vi "Calculate Duty Cycle.vi"(0 "Voltage/Current Values":dbl[](array[numeric]), 5 "Pulse voltage/Current level":dbl=1.0, 7 "Sample rate":dbl, 9 "Frequency":dbl, 11 "error in":errorcluster) -> (4 "Duty Cycle":dbl, 15 "error out":errorcluster)   [LabVIEW 2021]
doc: "This VI calculates the duty cycle high percentage using the rising and falling thresholds of current/voltage vaules."
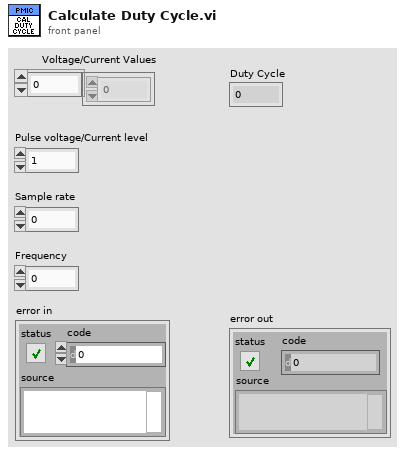
[diagram p1: front panel]
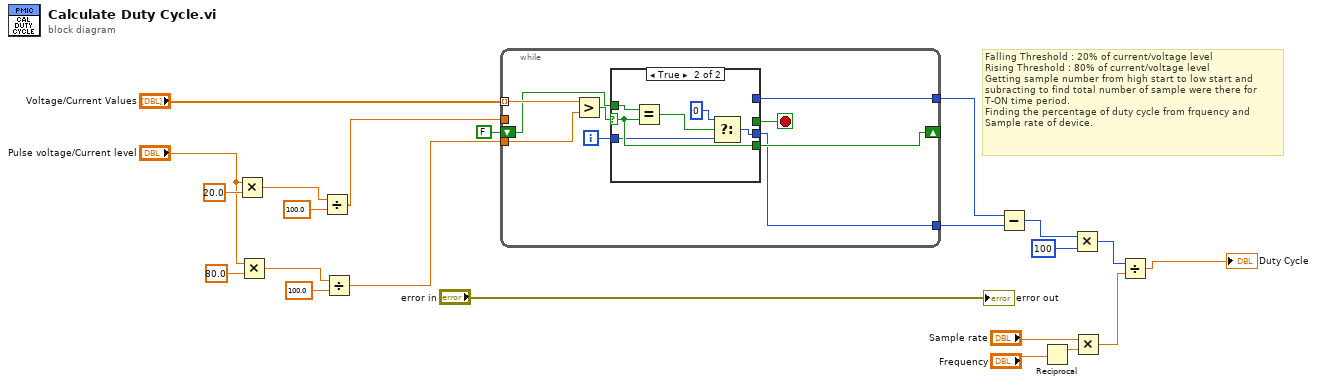
[diagram p0: block diagram]
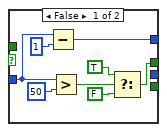
[diagram p2: hidden frame]
diagram:
  # "Falling Threshold : 20% of current/voltage level\nRising Threshold : 80% of current/voltage level\nGetting sample number from high start to low start and \nsubracting to find total number of sample were there for\nT-ON time period.\nFinding the percentage of duty cycle from frquency and\nSample rate of device."
  n1 = Multiply(x="Pulse voltage/Current level", y=20.0) -> (x*y=w21:dbl)
  n2 = Multiply(x="Pulse voltage/Current level", y=80.0) -> (x*y=w18:dbl)
  n3 = Divide(x=w21, y=100.0) -> (x/y=w6:dbl)
  n4 = Divide(x=w18, y=100.0) -> (x/y=w7:dbl)
  n5 = while {
    tunnel: "Voltage/Current Values" -> [w30] mode=indexing
    tunnel: w6 -> [_]
    tunnel: w7 -> [w31]
    shift-right: [w27] -> _
    shift-left: FALSE -> [w26]
    tunnel: [w25] -> w3
    tunnel: [w24] -> w4
    i -> [w28]
    stop <- w23 stop-if-true
    n6 = Greater?(x=w30, y=w31) -> (0:w29:bool)
    n7 = case shown="True" w29 {
      selector: w29 -> [_ w45]
      tunnel: w28 -> [w32 w42]
      tunnel: [_ w45] -> w27
      tunnel: w26 -> [_ w44]
      tunnel: [_ w40] -> w25
      tunnel: [w38 _] -> w24
      tunnel: [w36 _] -> w23
      frame False {
        n8 = Subtract(x=w32, y=1) -> (x-y=w38:i32)
        n9 = Greater?(x=w32, y=50) -> (0:w34:bool)
        n10 = Select(t=TRUE, s=w34, f=FALSE) -> (s? t:f=w36:bool)
      }
      frame True {
        n11 = Equal?(x=w44, y=w45) -> (x = y?=w43:bool)
        n12 = Select(t=0, s=w43, f=w42) -> (s? t:f=w40:i32)
      }
    }
  }
  n13 = Subtract(x=w4, y=w3) -> (x-y=w15:i32)
  n14 = Reciprocal(x="Frequency") -> (1/x=w10:dbl)
  n15 = Multiply(x=w15, y=100) -> (x*y=w14:i32)
  n16 = Multiply(x="Sample rate", y=w10) -> (x*y=w13:dbl)
  n17 = Divide(x=w14, y=w13) -> (x/y=→"Duty Cycle":dbl)
  "error out" <- "error in"
